vi "Main_고전압동작검사.vi"(8 "error in (no error)":errorcluster) -> (0 "error out":errorcluster)   [LabVIEW 2019]
uses:
  common/Sample Check.ctl
panel:
  in  "Tab Control":T1
  out "Pre Charge Relay 6":T2
  out "Pre Charge Relay 5":T2
  out "Pre Charge Relay 4":T2
  out "Pre Charge Relay 3":T2
  out "Pre Charge Relay 2":T2
  out "Pre Charge Relay 1":T2
  out "Waveform Graph 6":dbl[](graph)
  out "Waveform Graph 5":dbl[](graph)
  out "Waveform Graph 4":dbl[](graph)
  out "Waveform Graph 3":dbl[](graph)
  out "Waveform Graph 2":dbl[](graph)
  out "Waveform Graph":dbl[](graph)
  in  "고장진단 기준 값":T4
  in  "캐패시터부하":T5
  in  "파일 생성 주기[N]":dbl
  in  "저장 경로":path
  in  "시험명":string
  in  "그래프":bool
  in  "Main":bool
  in  "정지":bool
  in  "시작":bool
  in  "RESET":bool
  in  "시험세팅":bool
  in  "stop":bool
  in  "Enqueue Element":bool
  # "Pre Charge Relay 환경메카 신뢰성_고전압동작검사"
  # "Pre Charge Relay #1"
  # "Pre Charge Relay #4"
  # "Pre Charge Relay #2"
  # "Pre Charge Relay #5"
  # "Pre Charge Relay #3"
  # "Pre Charge Relay #6"
  # "Pre Charge Relay #1"
  # "Pre Charge Relay #4"
  # "Pre Charge Relay #2"
  # "Pre Charge Relay #5"
  # "Pre Charge Relay #3"
  # "Pre Charge Relay #6"
  # "제어단"
  # "출력단"
  # "부하전압 허용치(출력 파워서플라이 세팅 레벨 기준)"
  # "온도 기준"
  # "<=   측정 전류 값   <="
  # ">=   측정 전류 값"
  # "<=   측정 전류 값"
  # "<=   측정 전류 값   <="
  # ">=   측정 전류 값"
  # "<=   측정 전류 값"
  # "고전압"
  # "충전기준"
  # "제어전압"
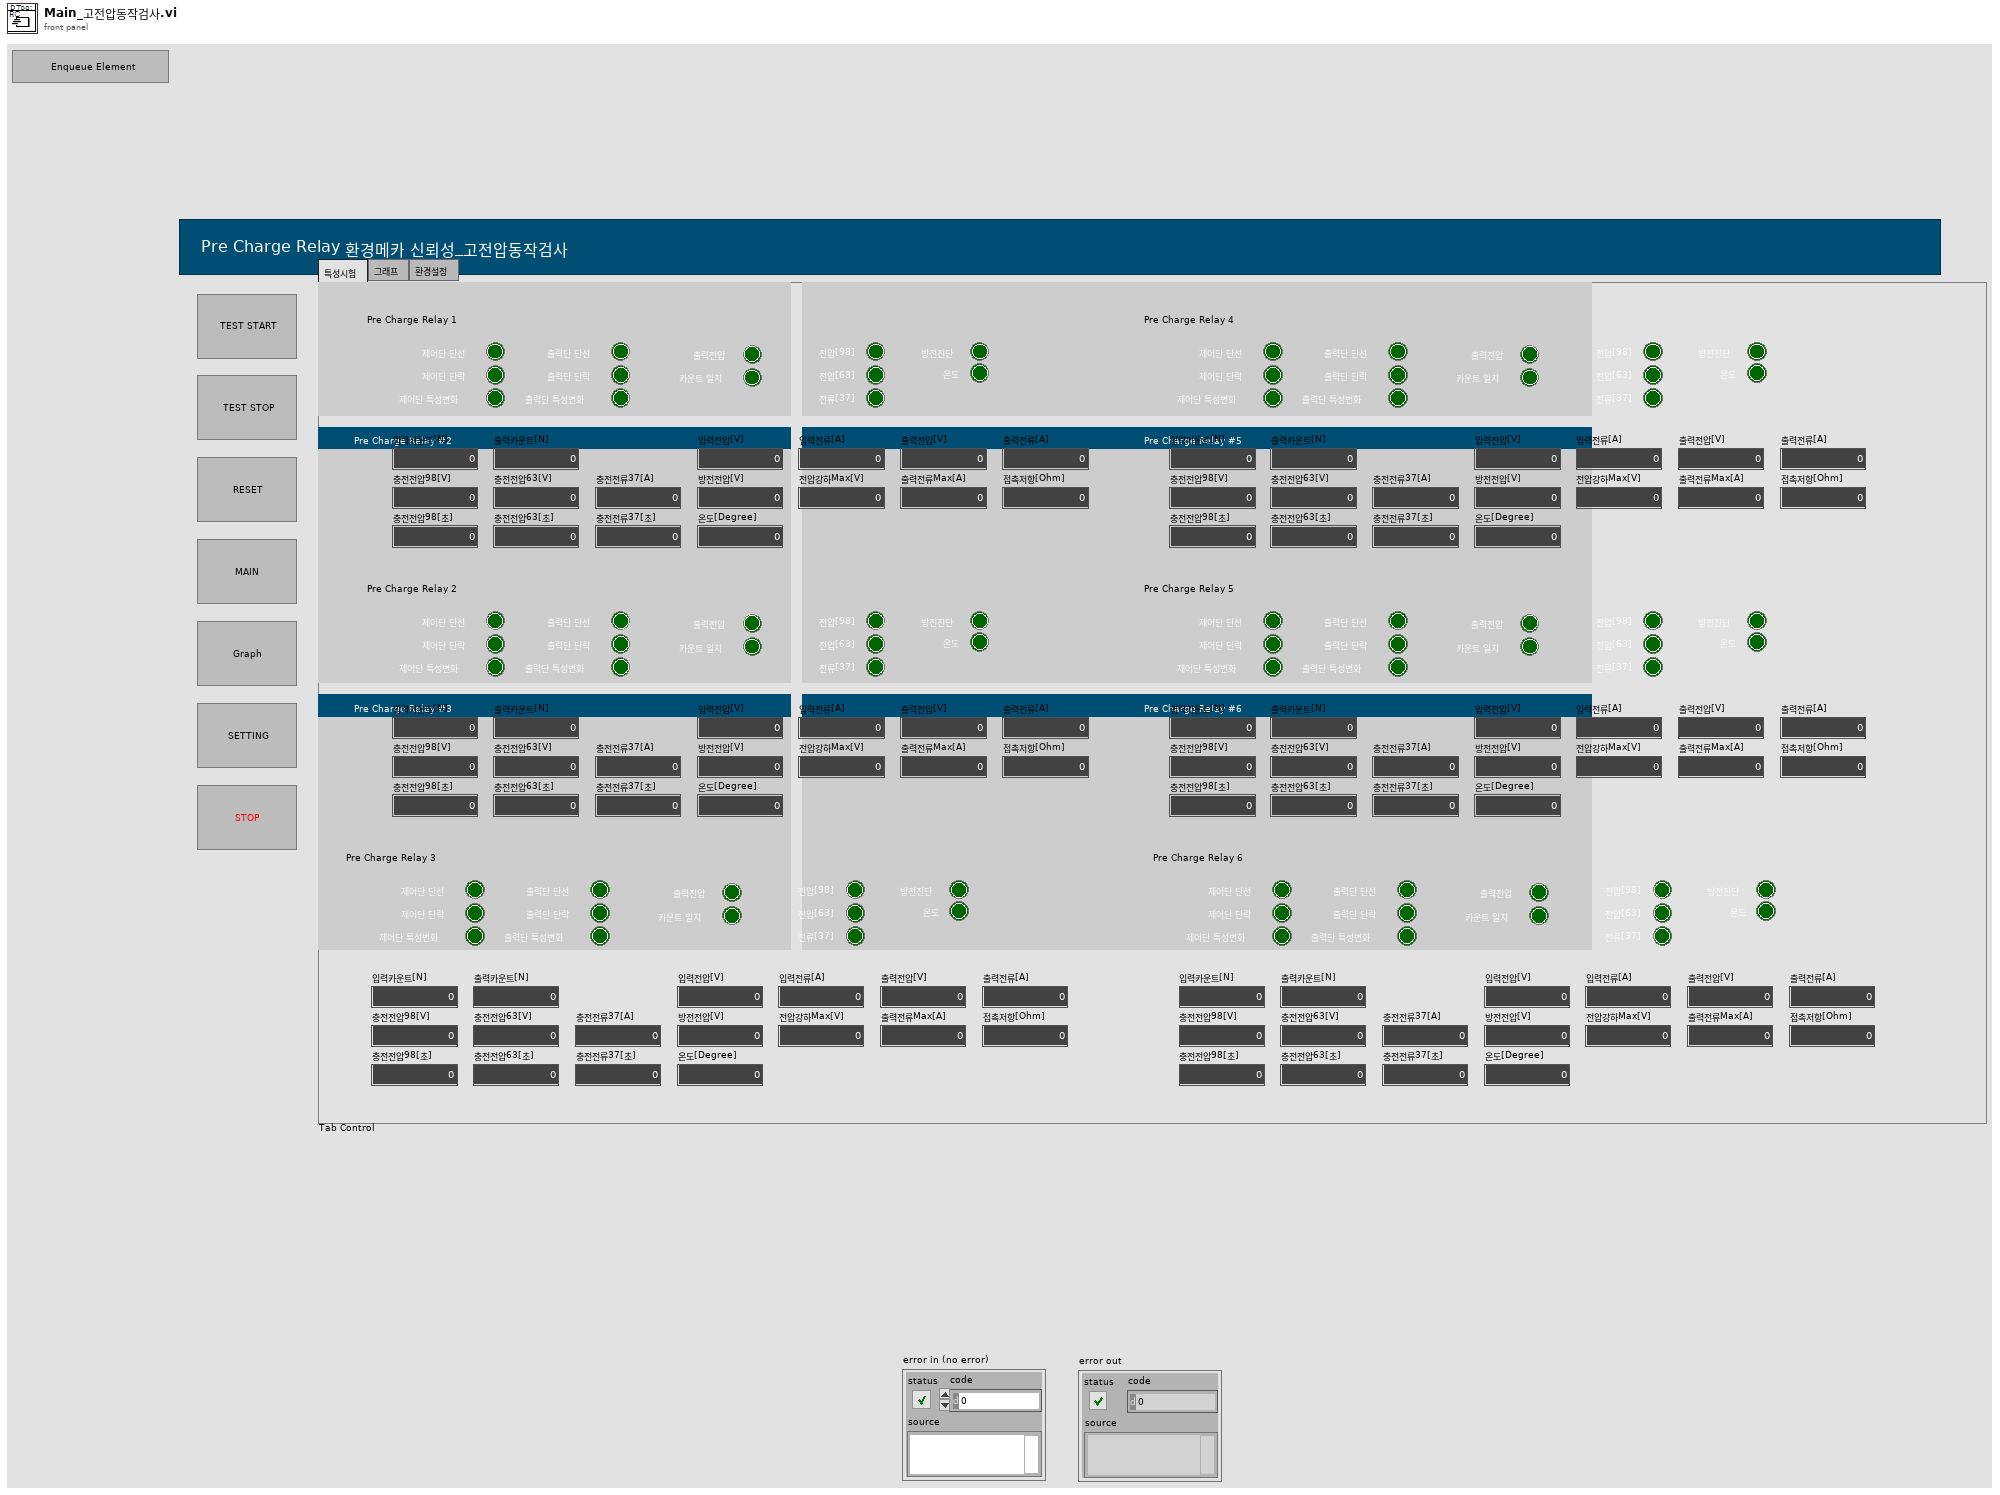
[diagram p1: front panel]
types:
  T1 = typedef "Tap_환경시험.ctl" = enum32{"특성시험", "그래프", "환경설정"}
  T2 = typedef "Data_고전압동작검사.ctl" = cluster{"입력카운트[N]":dbl, "출력카운트[N]":dbl, "입력전압[V]":dbl, "입력전류[A]":dbl, "출력전압[V]":dbl, "출력전류[A]":dbl, "충전전압98[V]":dbl, "충전전압63[V]":dbl, "충전전류37[A]":dbl, "방전전압[V]":dbl, "전압강하Max[V]":dbl, "출력전류Max[A]":dbl, "접촉저항[Ohm]":dbl, "충전전압98[초]":dbl, "충전전압63[초]":dbl, "충전전류37[초]":dbl, "제어단 단선":T3, "제어단 단락":T3, "제어단 특성변화":T3, "출력단 단선":T3, "출력단 단락":T3, "출력단 특성변화":T3, "카운트 일치":T3, "전압[98]":T3, "전압[63]":T3, "전류[37]":T3, "방전진단":T3, "출력전압":T3, "온도":T3, "온도[Degree]":dbl}
  T3 = typedef "Sample Check.ctl" = enum32{"idle", "OK", "NG", "Test"}
  T4 = typedef "공통_환경 진단모드.ctl" = cluster{"제어단 단선[A]":dbl, "제어단 단락[A]":dbl, "제어단 특성변화[A] From":dbl, "제어단 특성변화[A] to":dbl, "출력단 단선[A]":dbl, "출력단 단락[A]":dbl, "출력단 특성변화[A] From":dbl, "출력단 특성변화[A] to":dbl, "부하전압[+/-%] ":dbl, "측정온도[Degree] ":dbl}
  T5 = typedef "세팅_고전압동작검사.ctl" = cluster{"제어 전압[V]":dbl, "출력전압[V]":dbl, "전류[A]":dbl, "출력전류[A]":dbl, "ON[초]":dbl, "OFF[초]":dbl, "시험횟수[N]":dbl, "방전 진단[V]":dbl, "전압98[초]":dbl, "전압63[초]":dbl, "전류37[초]":dbl, "방전 시간[초]":dbl, "전압98[+/-%]":dbl, "전압63[+/-%]":dbl, "전류37[+/-%]":dbl}
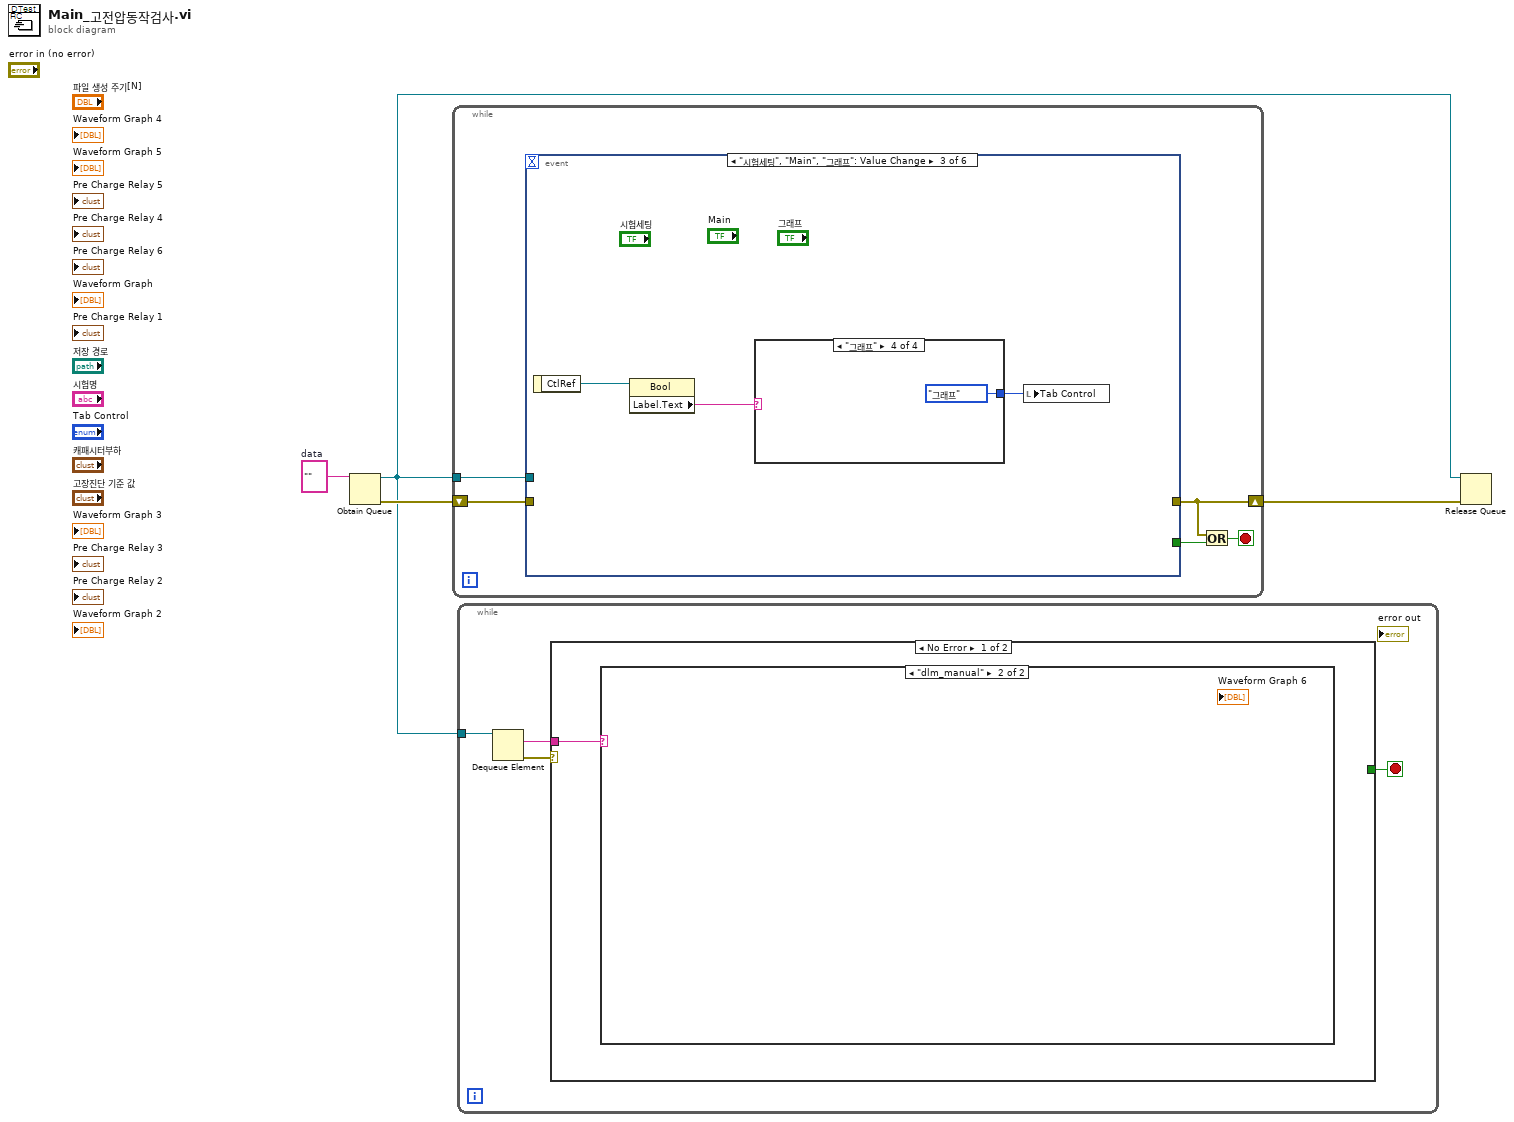
[diagram p0: block diagram]
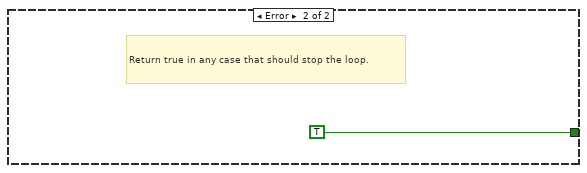
[diagram p3: hidden frame]
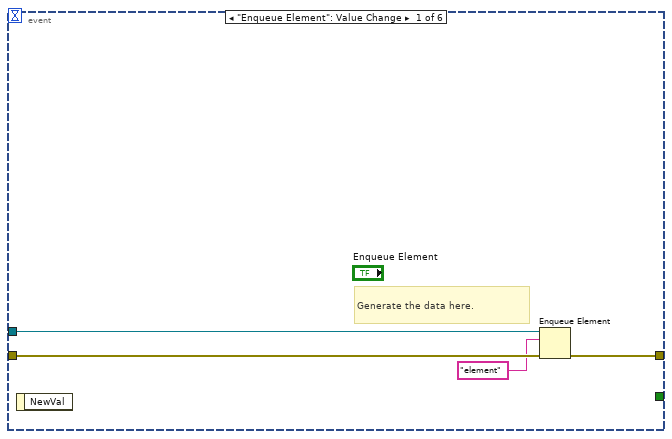
[diagram p4: hidden frame]
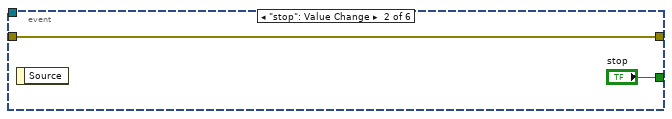
[diagram p5: hidden frame]
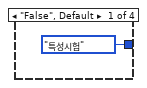
[diagram p6: hidden frame]
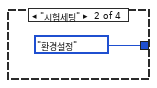
[diagram p7: hidden frame]
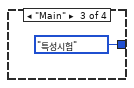
[diagram p8: hidden frame]
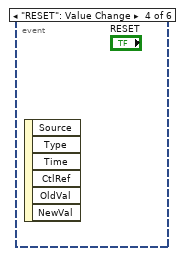
[diagram p9: hidden frame]
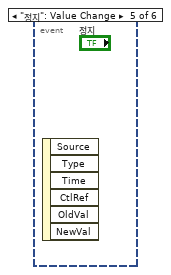
[diagram p10: hidden frame]
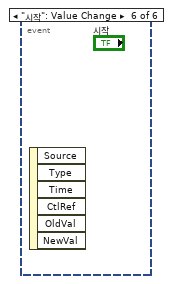
[diagram p11: hidden frame]
diagram:
  w2 = ""  # data
  n1 = Obtain Queue(element data type=w2) -> (queue out=w1:refnum<queue>, error out=w4:errorcluster)  [unwired: 4 in, 1 out]
  n2 = while {
    shift-right: [w5] -> w3
    shift-left: w4 -> [w8]
    tunnel: w1 -> [w9]
    stop <- w6 stop-if-true
    n3 = event shown="[2] \"시험세팅\", \"Main\", \"그래프\": Value Change" {
      selector: _ -> [_ _ _ _ _ _]
      dyn-events: _ -> [_ _ _ _ _ _]
      timeout: _ -> [_ _ _ _ _ _]
      tunnel: w9 -> [w13 _ _ _ _ _]
      tunnel: w8 -> [w12 w14 _ _ _ _]
      tunnel: [w11 w14 _ _ _ _] -> w5
      tunnel: [_ "stop" _ _ _ _] -> w7
      event "Enqueue Element": Value Change {
        # "Generate the data here."
        n4 = event-data() -> ()  [unwired: 1 in, 1 out]
        n5 = Enqueue Element(queue=w13, element="element", error in (no error)=w12) -> (error out=w11:errorcluster)  [unwired: 1 in, 2 out]
      }
      event "stop": Value Change {
        n6 = event-data() -> ()  [unwired: 1 in, 1 out]
      }
      event "시험세팅", "Main", "그래프": Value Change {
        n7 = event-data() -> ("CtlRef"=w18:refnum<vi>)  [unwired: 1 in]
        n8 = property class="Bool"(reference=w18) -> ("Label.Text"=w17:string)  [unwired: 1 in, 2 out]
        n9 = case shown="\"그래프\"" w17 {
          tunnel: [Tap_환경시험."특성시험" ("Tab Control") Tap_환경시험."환경설정" ("Tab Control") Tap_환경시험."특성시험" ("Tab Control") Tap_환경시험."그래프" ("Tab Control")] -> w16
          frame "False", Default {
          }
          frame "시험세팅" {
          }
          frame "Main" {
          }
          frame "그래프" {
          }
        }
        n10 = local write "Tab Control"(w16) -> ()
      }
      event "RESET": Value Change {
        n11 = event-data() -> ()  [unwired: 1 in, 6 out]
      }
      event "정지": Value Change {
        n12 = event-data() -> ()  [unwired: 1 in, 6 out]
      }
      event "시작": Value Change {
        n13 = event-data() -> ()  [unwired: 1 in, 6 out]
      }
    }
    n14 = Or(x=w5, y=w7) -> (x .or. y?=w6:bool)
  }
  n15 = while {
    tunnel: w1 -> [w26]
    stop <- w23 stop-if-true
    n16 = Dequeue Element(queue=w26) -> (element=w24:string, error out=w25:errorcluster)  [unwired: 2 in, 2 out]
    n17 = case shown="No Error" w25 {
      tunnel: w24 -> [w27 _]
      tunnel: [_ TRUE] -> w23
      frame No Error {
        n18 = case shown="\"dlm_manual\"" w27 {
          frame "False", Default {
          }
          frame "dlm_manual" {
          }
        }
      }
      frame Error {
        # "Return true in any case that should stop the loop."
      }
    }
  }
  n19 = Release Queue(queue=w1, error in (no error)=w3) -> ()  [unwired: 1 in, 3 out]
